vi "Get Number HS Speeds.vi"(9 "speeds":i32, 10 "typ":i32, 11 "channel":i32) -> (1 "speeds out":i32, 3 "function return":u32)   [LabVIEW 2018, in "AndorSDK.lvlib"]
doc: "EXPNETTYPE unsigned int WINAPI GetNumberHSSpeeds(int channel, int typ, int * speeds);"
uses:
  AndorSDK.lvlib
  ATMCD32D.dll
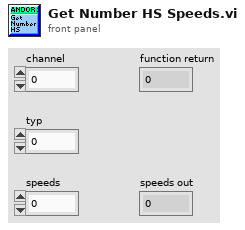
[diagram p1: front panel]
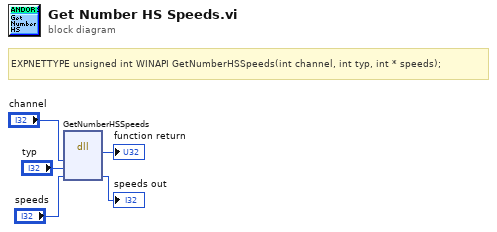
[diagram p0: block diagram]
diagram:
  # "EXPNETTYPE unsigned int WINAPI GetNumberHSSpeeds(int channel, int typ, int * speeds);"
  n1 = dll-call lib="PTH2babs E\nPersönliches02 - Arbeit03-HiwijobsLabviewCodelibANDOR\tAndor SDK\nATMCD32D.*" fn="GetNumberHSSpeeds"("channel"="channel", "typ"="typ", "speeds"="speeds") -> (→"function return":u32, "speeds"=→"speeds out":i32)  [unwired: 5 in, 2 out]
